vi "Get Object Torrent.vi"(4 "Region":T1, 8 "error in (no error)":errorcluster, 9 "Bucket":string, 10 "Object Path":string, 11 "Torrent file path":path=path "") -> (0 "error out":errorcluster, 3 "Torrent file data (RAW)":string)   [LabVIEW 2015, in "LV Interface for Amazon S3.lvlib"]
doc: "This operation <B>returns torrent files from a bucket</B>. BitTorrent can save you bandwidth when you're distributing large files. <B>Note:</B> You can <B>get torrent only for objects</B> that are <B>less than 5 GB</> in size. You must have READ access</B> to the object."
uses:
  LV Interface for Amazon S3.lvlib
  Typedefs/AMZ_S3_LocationConstraint.ctl
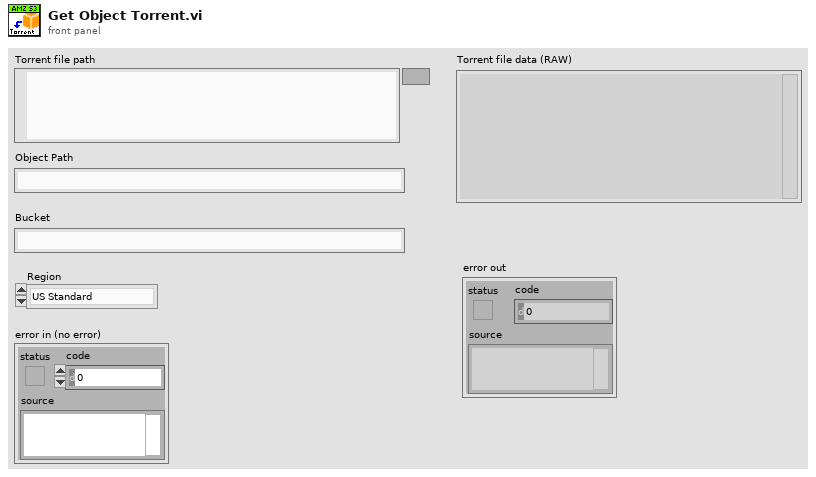
[diagram p1: front panel]
types:
  T1 = typedef "LV Interface for Amazon S3.lvlib/AMZ_S3_LocationConstraint.ctl" = enum16{"US Standard", "us-east-2", "us-west-1", "us-west-2", "ap-northeast-1", "ap-northeast-2", "ap-southeast-1", "ap-southeast-2", "ca-central-1", "eu-central-1", "eu-west-1", "eu-west-2", "sa-east-1"}
  T2 = enum16{"open", "replace", "create", "open or create", "replace or create", "replace or create with confirmation"}
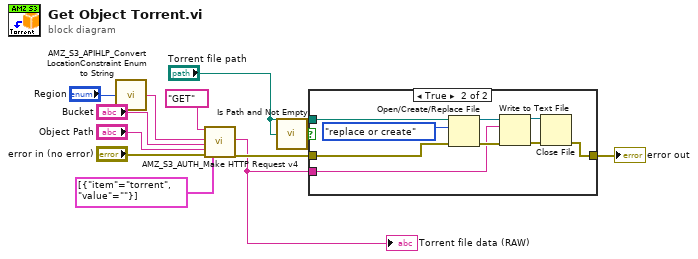
[diagram p0: block diagram]
diagram:
  n1 = call "AMZ_S3_APIHLP_Convert LocationConstraint Enum to String.vi"("Location"="Region") -> ("Location String"=w1:string)  [unwired: 4 in]
  n2 = call "AMZ_S3_AUTH_Make HTTP Request v4.vi"("HTTP-Verb"="GET", "Region"=w1, "Bucket"="Bucket", "Object Key"="Object Path", "error in"="error in (no error)", "request parameters"=cluster{"item":string, "value":string}[] [{"item"="torrent", "value"=""}]) -> ("response body"=w3:string, "error out"=w6:errorcluster)  [unwired: 10 in, 2 out]
  "Torrent file data (RAW)" <- w3
  n3 = call <vilib>:"Is Path and Not Empty.vi"("path"="Torrent file path") -> ("Is Path and Not Empty?"=w5:bool)  [unwired: 4 in]
  n4 = case shown="True" w5 {
    tunnel: "Torrent file path" -> [_ w22]
    tunnel: w6 -> [w13 w21]
    tunnel: [w13 w15] -> w4
    tunnel: w3 -> [_ w19]
    frame False {
    }
    frame True {
      n5 = Open/Create/Replace File(file path (use dialog)=w22, error in=w21, operation (0:open)=T2."replace or create") -> (refnum out=w18:refnum<file>, error out=w20:errorcluster)  [unwired: 3 in, 1 out]
      n6 = Write to Text File(file (use dialog)=w18, text=w19, error in=w20) -> (refnum out=w16:refnum<file>, error out=w17:errorcluster)  [unwired: 1 in, 1 out]
      n7 = Close File(refnum=w16, error in=w17) -> (error out=w15:errorcluster)  [unwired: 1 out]
    }
  }
  "error out" <- w4
